vi "gds_modulate.vi"(8 "error in (no error)":errorcluster, 10 "input bit stream":i8[](array[numeric]), 11 "Modulation Parameters":T1) -> (0 "error out":errorcluster, 1 "symbols out":cdb[](array[numeric]) format="%.2f", 2 "output complex waveform":T2 {"Y" format="%.3f"; "dt" format="%^.2e"; "t0" format="%.4f"}, 3 "Modulation Parameters  Out":T1)   [LabVIEW 2012]
uses:
  <vilib>/addons/Modulation/Analog/controls/Complex Data Waveform.ctl
  <vilib>/addons/Modulation/Digital/General/MT Generate FSK System Parameters(M).vi
  <vilib>/addons/Modulation/Digital/General/MT Generate ASK system parameters (M).vi
  <vilib>/addons/Modulation/niDMT.lvlib
  <vilib>/addons/Modulation/niAMT.lvlib
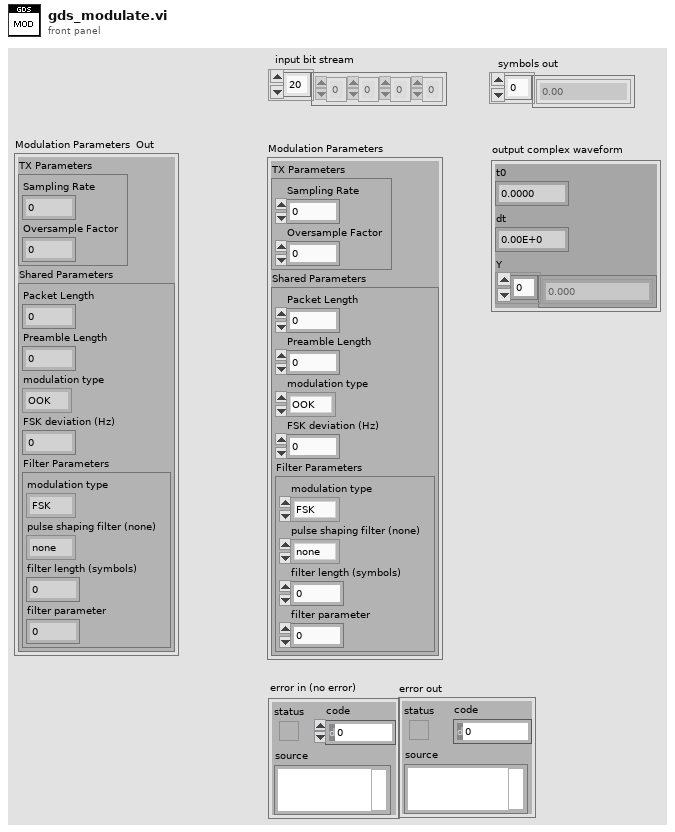
[diagram p1: front panel]
types:
  T1 = cluster{"TX Parameters":cluster{"Sampling Rate":dbl, "Oversample Factor":i32}, "Shared Parameters":cluster{"Packet Length":i32, "Preamble Length":i32, "modulation type":enum16{"OOK", "FSK", "PSK", "QAM", "MSK", "PAM", "ASK", "CPM"}, "FSK deviation (Hz)":dbl, "Filter Parameters":cluster{"modulation type":enum16{"FSK", "PSK", "QAM", "MSK", "PAM", "ASK", "CPM"}, "pulse shaping filter (none)":enum16{"none", "Raised Cosine", "Root Raised Cos", "Gaussian"}, "filter length (symbols)":i32, "filter parameter":dbl}}}
  T2 = typedef "niAMT.lvlib/Complex Data Waveform.ctl" = cluster{"t0":dbl, "dt":dbl, "Y":cdb[]}
  T3 = enum16{"OOK", "FSK", "PSK", "QAM", "MSK", "PAM", "ASK", "CPM"}
  T4 = enum16{"FSK", "PSK", "QAM", "MSK", "PAM", "ASK", "CPM"}
  T5 = enum16{"none", "Raised Cosine", "Root Raised Cos", "Gaussian"}
  T6 = cluster{"samples per symbol (16)":i32, "symbol map":dbl[], "symbol phase continuity":enum16{"continuous", "discontinuous"}}
  T7 = cluster{"samples per symbol (16)":i32, "symbol map":cdb[]}
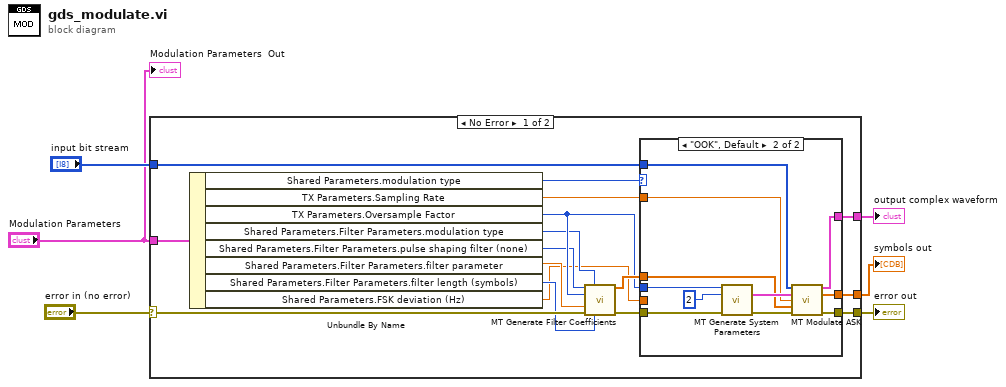
[diagram p0: block diagram]
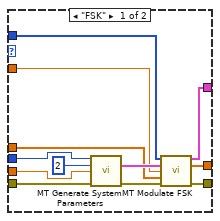
[diagram p2: hidden frame]
diagram:
  n1 = case shown="No Error" "error in (no error)" {
    selector: "error in (no error)" -> [w18 w46]
    tunnel: [w22 _] -> w6
    tunnel: [w21 w46] -> w4
    tunnel: [w20 _] -> w3
    tunnel: "input bit stream" -> [w19 _]
    tunnel: "Modulation Parameters" -> [w15 _]
    frame No Error {
      n2 = Unbundle By Name(w15) -> ("Shared Parameters.modulation type"=w8:T3, "TX Parameters.Sampling Rate"=w14:dbl, "TX Parameters.Oversample Factor"=w13:i32, "Shared Parameters.Filter Parameters.modulation type"=w12:T4, "Shared Parameters.Filter Parameters.pulse shaping filter (none)"=w11:T5, "Shared Parameters.Filter Parameters.filter parameter"=w10:dbl, "Shared Parameters.Filter Parameters.filter length (symbols)"=w9:i32, "Shared Parameters.FSK deviation (Hz)"=w7:dbl)
      n3 = call <vilib>:"MT Generate Filter Coefficients.vi"("pulse shaping filter (none)"=w11, "modulation type"=w12, "pulse shaping samples per symbol (16)"=w13, "filter parameter"=w10, "error in (no error)"=w18, "filter length (symbols)"=w9) -> ("pulse shaping filter coefficients"=w16:dbl[], "error out"=w17:errorcluster)  [unwired: 7 in, 1 out]
      n4 = case shown="\"OOK\", Default" w8 {
        tunnel: [w28 w44] -> w22
        tunnel: [w26 w43] -> w21
        tunnel: [w27 w42] -> w20
        tunnel: w19 -> [w29 w41]
        tunnel: w14 -> [w24 w40]
        tunnel: w13 -> [w30 w39]
        tunnel: w17 -> [w31 w38]
        tunnel: w16 -> [w25 w36]
        tunnel: w7 -> [w23 _]
        frame "FSK" {
          n5 = call-poly <vilib>:"MT Generate System Parameters.vi"("samples per symbol (16)"=w30, "M-FSK (2)"=2 ("M-ASK (2)"), "FSK deviation (Hz)"=w23, "error in (no error)"=w31) -> ("FSK system parameters"=w34:T6, "error out"=w33:errorcluster)  [unwired: 9 in, 1 out]
          n6 = call <vilib>:"MT Modulate FSK.vi"("input bit stream"=w29, "FSK system parameters"=w34, "symbol rate (Hz)"=w24, "pulse shaping filter coefficients"=w25, "error in (no error)"=w33) -> ("output complex waveform"=w28:T2, "symbols out"=w27:dbl[], "error out"=w26:errorcluster)  [unwired: 8 in]
        }
        frame "OOK", Default {
          n7 = call-poly <vilib>:"MT Generate System Parameters.vi"("samples per symbol (16)"=w39, "M-ASK (2)"=2, "error in (no error)"=w38) -> ("ASK system parameters"=w45:T7, "error out"=w37:errorcluster)  [unwired: 10 in, 1 out]
          n8 = call <vilib>:"MT Modulate ASK.vi"("input bit stream"=w41, "ASK system parameters"=w45, "symbol rate (Hz)"=w40, "pulse shaping filter coefficients"=w36, "error in (no error)"=w37) -> ("output complex waveform"=w44:T2, "symbols out"=w42:cdb[], "error out"=w43:errorcluster)  [unwired: 8 in]
        }
      }
    }
    frame Error {
    }
  }
  "output complex waveform" <- w6
  "error out" <- w4
  "symbols out" <- w3
  "Modulation Parameters  Out" <- "Modulation Parameters"
